vi "delete_table.vi"(8 "error in (no error)":errorcluster, 10 "table_name":string, 11 "Doc in":refnum<class "Doc.lvclass">) -> (0 "error out":errorcluster, 2 "deleted?":bool, 3 "Doc out":refnum<class "Doc.lvclass">)   [LabVIEW 2020, in "toml_edit.lvlib" / "Doc.lvclass"]
uses:
  Doc.lvclass
  Doc.lvclass/Doc.ctl
  dragon_toml_64.dll
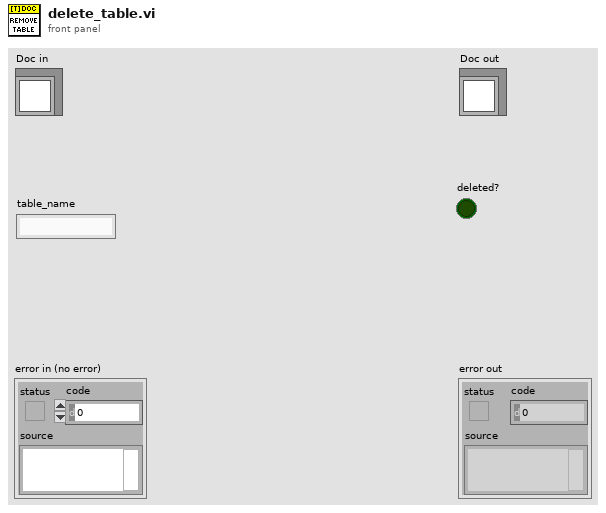
[diagram p1: front panel]
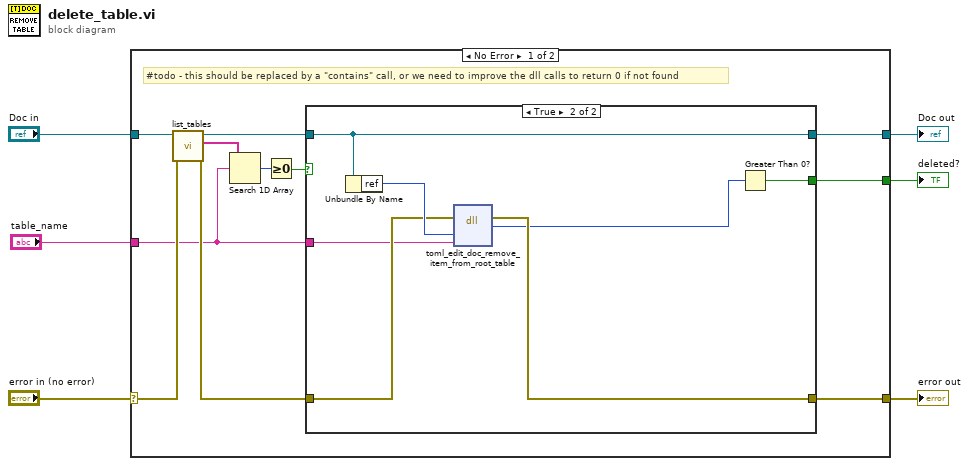
[diagram p0: block diagram]
diagram:
  n1 = case shown="No Error" "error in (no error)" {
    selector: "error in (no error)" -> [w14 w28]
    tunnel: [w17 w28] -> w5
    tunnel: [w8 w27] -> w3
    tunnel: "Doc in" -> [w15 w27]
    tunnel: "table_name" -> [w11 _]
    tunnel: [w7 _] -> w1
    frame No Error {
      # "#todo - this should be replaced by a \"contains\" call, or we need to improve the dll calls to return 0 if not found"
      n2 = call "list_tables.vi"("error in (no error)"=w14, "Doc in"=w15) -> ("error out"=w13:errorcluster, "table_names"=w12:string[], "Doc out"=w16:refnum<class "Doc.lvclass">)  [unwired: 7 in]
      n3 = Search 1D Array(1D array=w12, element=w11) -> (index of element=w10:i32)  [unwired: 1 in]
      n4 = Greater Or Equal To 0?(x=w10) -> (x >= 0?=w9:bool)
      n5 = case shown="True" w9 {
        tunnel: [w18 w25] -> w17
        tunnel: w16 -> [w19 w22]
        tunnel: w13 -> [w18 w24]
        tunnel: w11 -> [_ w23]
        tunnel: [w19 w22] -> w8
        tunnel: [_ w20] -> w7
        frame False {
        }
        frame True {
          n6 = Unbundle By Name(w22) -> ("ref"=w26:u64)
          n7 = dll-call lib="C:/projects/dragon-desktop/source/submodules/toml-edit-labview/lv_src/dragon_toml_*.dll" fn="toml_edit_doc_remove_item_from_root_table"(error in=w24, "doc_ref"=w26, "table_name"=w23) -> (error out=w25:errorcluster, "was_removed"=w21:u64)  [unwired: 4 in, 1 out]
          n8 = Greater Than 0?(x=w21) -> (x > 0?=w20:bool)
        }
      }
    }
    frame Error {
    }
  }
  "error out" <- w5
  "Doc out" <- w3
  "deleted?" <- w1
